vi "uc480_Flash_and_Trigger.vi"() -> ()   [LabVIEW 2016]
uses:
  D:/Fabrizio/Labview Projects/IR OPO Controller/Branches/Schwarzschild version/uc480DotNet.dll
  uc480DotNet.dll
panel:
  in  "Flash Duration":u32=10000
  in  "Flash Mode":string(combo)="0"
  in  "Trigger Mode":string(combo)="Software"
  out "Image":picture
  in  "Camera ID":i32 min=0 max=255
  out "Serial Number":string
  out "AOI Height":i32=8
  out "AOI Width":i32=8
  out "Bits/Pixel":i32=8
  out "Error Out":errorcluster caption="error"
  in  "Exit Camera":bool
  in  "Init Camera":bool
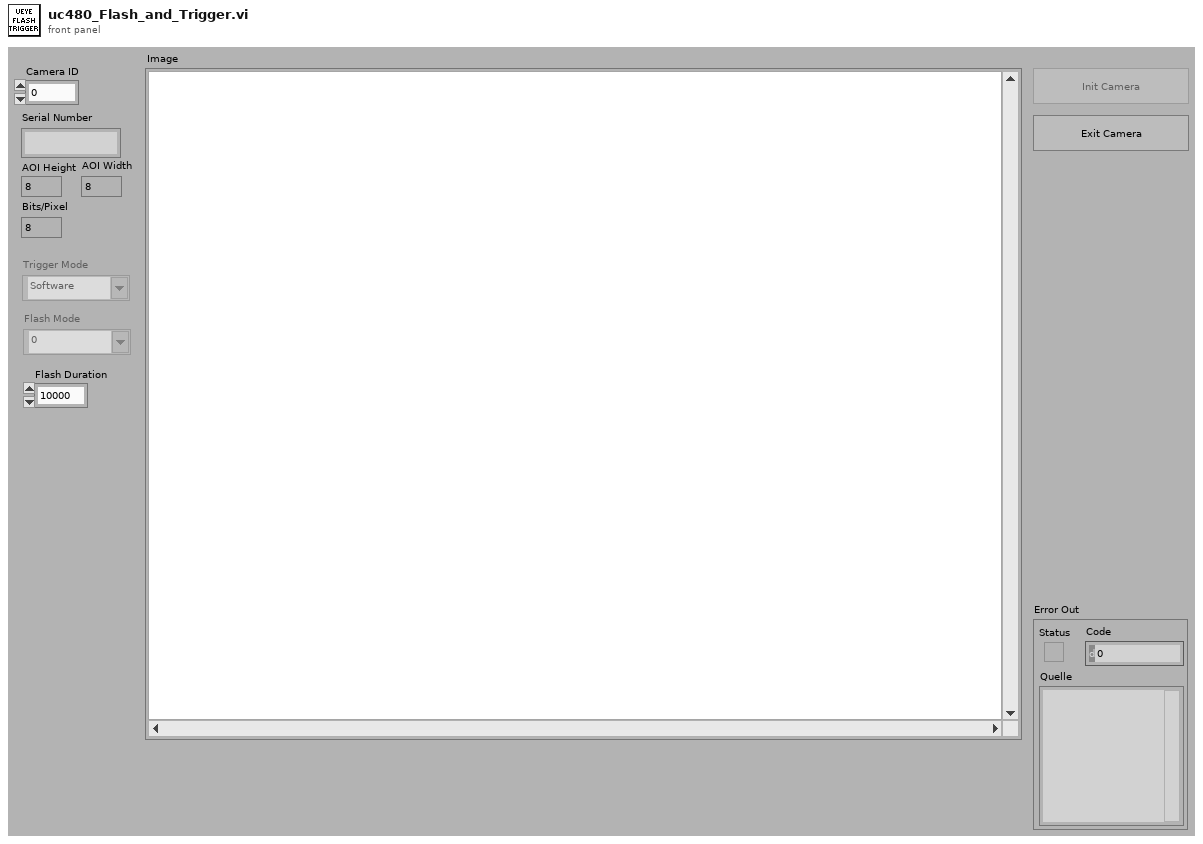
[diagram p1: front panel]
types:
  T1 = enum8{"Enabled", "Disabled", "Disabled and Grayed Out"}
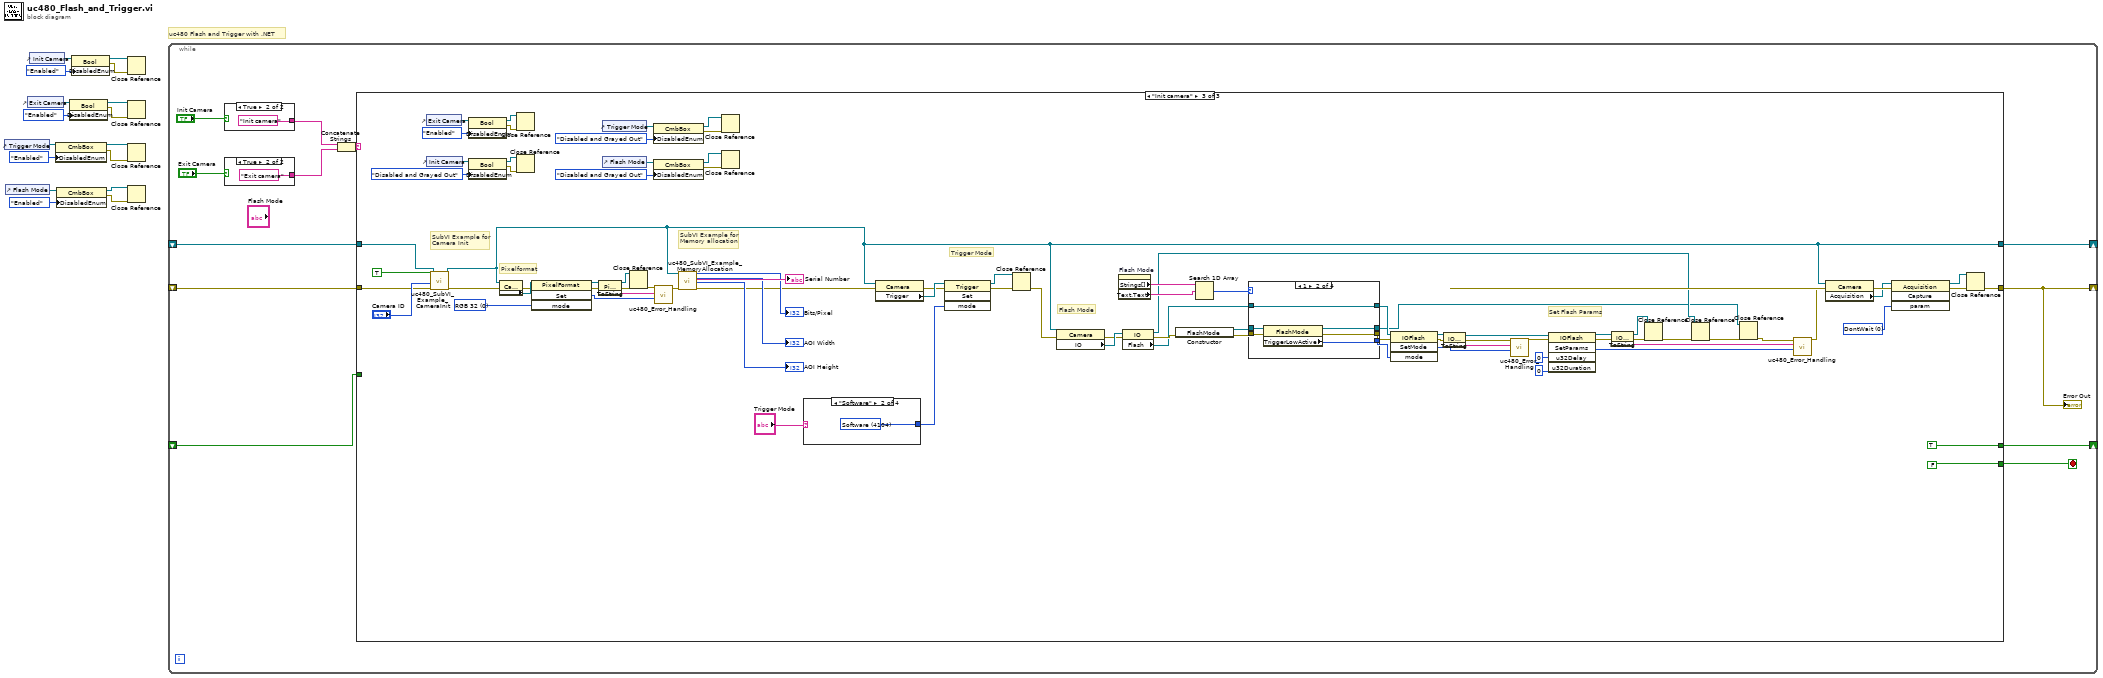
[diagram p0: block diagram]
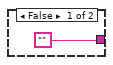
[diagram p2: hidden frame]
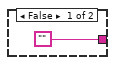
[diagram p3: hidden frame]
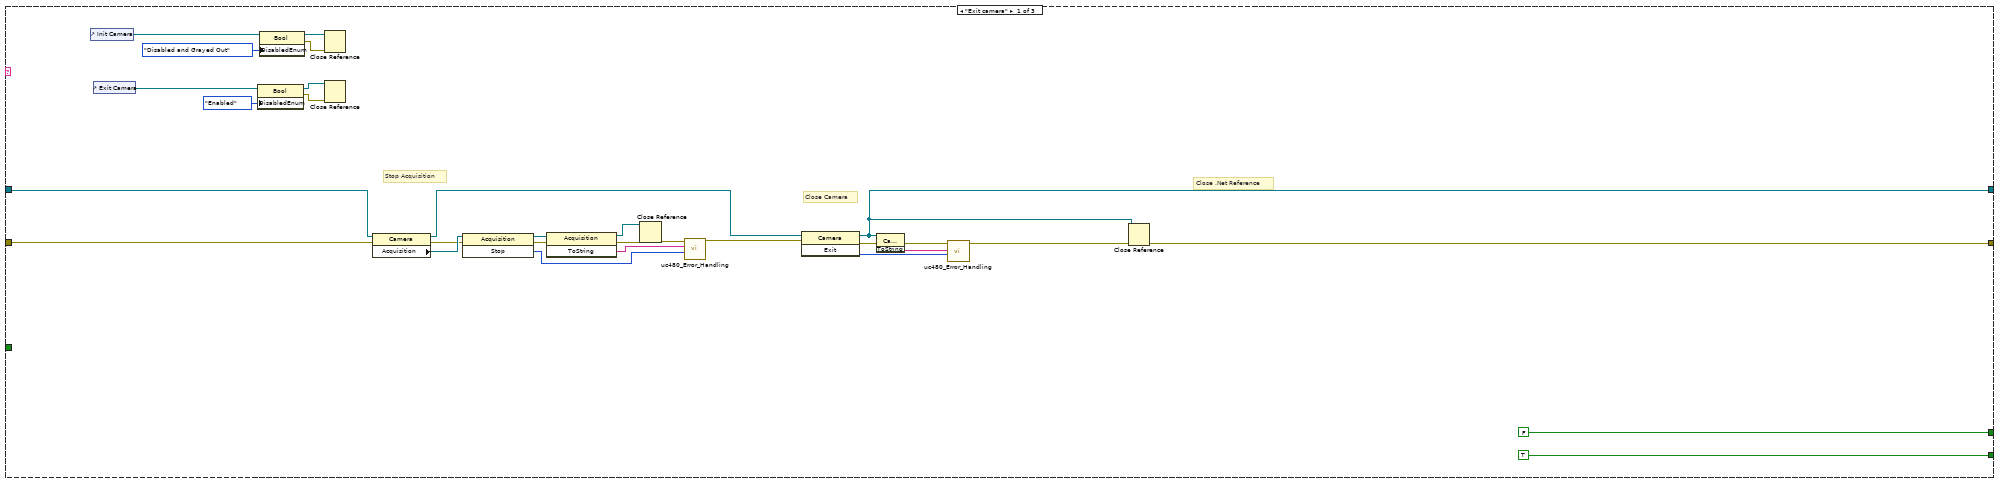
[diagram p4: hidden frame]
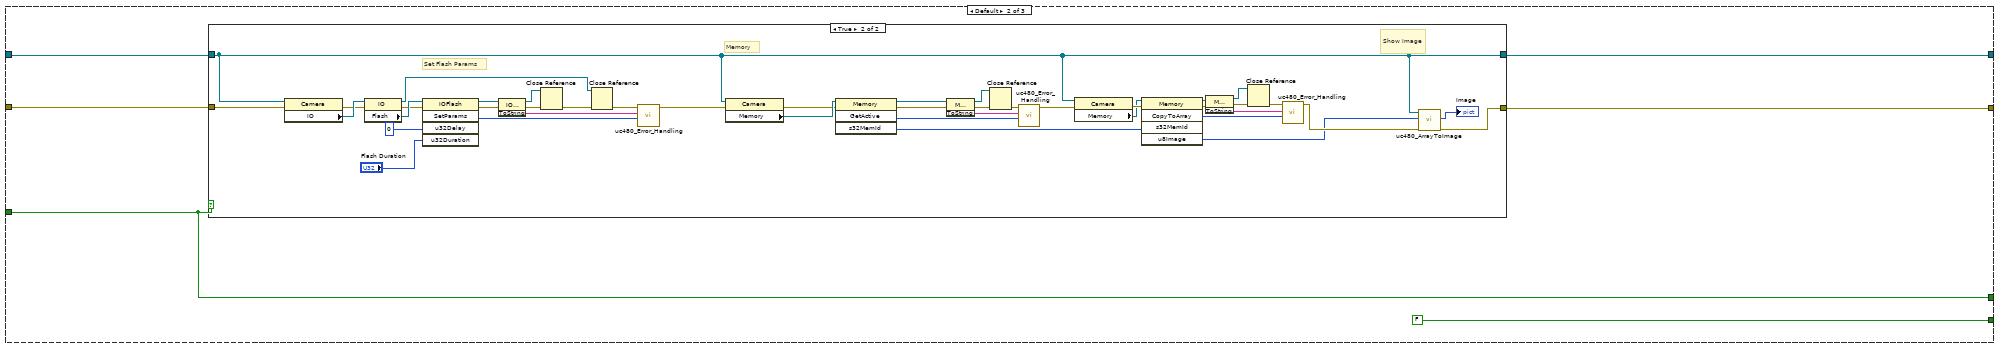
[diagram p5: hidden frame]
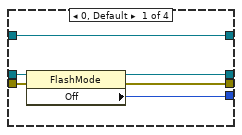
[diagram p7: hidden frame]
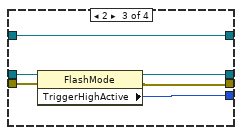
[diagram p8: hidden frame]
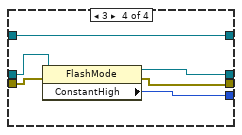
[diagram p9: hidden frame]
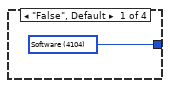
[diagram p10: hidden frame]
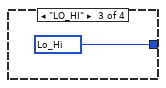
[diagram p11: hidden frame]
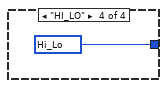
[diagram p12: hidden frame]
diagram:
  # "uc480 Flash and Trigger with .NET"
  n1 = control-ref of="Trigger Mode"() -> (w11:refnum<vi>)
  n2 = control-ref of="Flash Mode"() -> (w9:refnum<vi>)
  n3 = control-ref of="Exit Camera"() -> (w13:refnum<vi>)
  n4 = control-ref of="Init Camera"() -> (w14:refnum<vi>)
  n5 = property class="CmbBox"(reference=w11, "DisabledEnum"=T1."Enabled" ("Disabled")) -> (reference out=w5:refnum<vi>, error out=w6:errorcluster)  [unwired: 1 in]
  n6 = property class="CmbBox"(reference=w9, "DisabledEnum"=T1."Enabled" ("Disabled")) -> (reference out=w7:refnum<vi>, error out=w8:errorcluster)  [unwired: 1 in]
  n7 = property class="Bool"(reference=w13, "DisabledEnum"=T1."Enabled" ("Disabled")) -> (reference out=w3:refnum<vi>, error out=w4:errorcluster)  [unwired: 1 in]
  n8 = property class="Bool"(reference=w14, "DisabledEnum"=T1."Enabled" ("Disabled")) -> (reference out=w1:refnum<vi>, error out=w2:errorcluster)  [unwired: 1 in]
  n9 = Close Reference(reference=w1, error in (no error)=w2) -> ()  [unwired: 1 out]
  n10 = Close Reference(reference=w3, error in (no error)=w4) -> ()  [unwired: 1 out]
  n11 = Close Reference(reference=w5, error in (no error)=w6) -> ()  [unwired: 1 out]
  n12 = Close Reference(reference=w7, error in (no error)=w8) -> ()  [unwired: 1 out]
  n13 = while {
    shift-right: [w20] -> _
    shift-left: _ -> [w23]
    shift-right: [w22] -> _
    shift-left: _ -> [w17]
    shift-right: [w19] -> _
    shift-left: _ -> [w18]
    stop <- w21 stop-if-true
    n14 = case shown="True" "Init Camera" {
      tunnel: ["" "Init camera"] -> w27
      frame False {
      }
      frame True {
      }
    }
    n15 = case shown="True" "Exit Camera" {
      tunnel: ["" "Exit camera"] -> w24
      frame False {
      }
      frame True {
      }
    }
    n16 = Concatenate Strings(w27, w24) -> (w26:string)
    n17 = case shown="\"Init camera\"" w26 {
      tunnel: w17 -> [w38 w64 w190]
      tunnel: w23 -> [w47 w63 w189]
      tunnel: [w56 w66 w146] -> w22
      tunnel: [w55 w67 w128] -> w20
      tunnel: [TRUE FALSE FALSE] -> w21
      tunnel: [FALSE w65 TRUE] -> w19
      tunnel: w18 -> [_ w65 _]
      frame "Exit camera" {
        # "Close .Net Reference"
        # "Stop Acquisition"
        # "Close Camera"
        n18 = control-ref of="Init Camera"() -> (w43:refnum<vi>)
        n19 = control-ref of="Exit Camera"() -> (w42:refnum<vi>)
        n20 = property class="Bool"(reference=w42, "DisabledEnum"=T1."Enabled" ("Disabled")) -> (reference out=w33:refnum<vi>, error out=w34:errorcluster)  [unwired: 1 in]
        n21 = property class="Bool"(reference=w43, "DisabledEnum"=T1."Disabled and Grayed Out" ("Disabled")) -> (reference out=w35:refnum<vi>, error out=w36:errorcluster)  [unwired: 1 in]
        n22 = Close Reference(reference=w35, error in (no error)=w36) -> ()  [unwired: 1 out]
        n23 = Close Reference(reference=w33, error in (no error)=w34) -> ()  [unwired: 1 out]
        n24 = property class="Camera"(reference=w38, error in=w47) -> (reference out=w37:refnum<k24>, error out=w51:errorcluster, "Acquisition"=w52:refnum<k24>)
        n25 = invoke class="Acquisition" method="Stop"(reference=w52, error in=w51) -> (reference out=w49:refnum<k24>, error out=w50:errorcluster, "Stop"=w48:i32)  [unwired: 1 in]
        n26 = invoke class="Acquisition" method="ToString"(reference=w49, error in=w50) -> (reference out=w39:refnum<k24>, error out=w41:errorcluster, "ToString"=w53:string)  [unwired: 1 in]
        n27 = Close Reference(reference=w39, error in (no error)=w41) -> (error out=w40:errorcluster)
        n28 = call "uc480_Error_Handling.vi"("Error Code"=w48, "Error String"=w53, "Error In"=w40) -> ("Error Out"=w46:errorcluster)  [unwired: 8 in]
        n29 = invoke class="Camera" method="Exit"(reference=w37, error in=w46) -> (reference out=w56:refnum<k24>, error out=w59:errorcluster, "Exit"=w58:i32)  [unwired: 1 in]
        n30 = invoke class="Camera" method="ToString"(reference=w56, error in=w59) -> (error out=w60:errorcluster, "ToString"=w61:string)  [unwired: 1 in, 1 out]
        n31 = call "uc480_Error_Handling.vi"("Error Code"=w58, "Error String"=w61, "Error In"=w60) -> ("Error Out"=w57:errorcluster)  [unwired: 8 in]
        n32 = Close Reference ("Close Referenz")(reference=w56, error in (no error)=w57) -> (error out=w55:errorcluster)
      }
      frame Default {
        n33 = case shown="True" w65 {
          tunnel: [w70 w98] -> w67
          tunnel: w63 -> [w70 w83]
          tunnel: w64 -> [w69 w82]
          tunnel: [w69 w82] -> w66
          frame False {
          }
          frame True {
            # "Set Flash Params"
            # "Show Image"
            # "Memory"
            n34 = property on="Eigenschaftsknoten" class="Camera"(reference=w82, error in=w83) -> (error out=w89:errorcluster, "IO"=w91:refnum<k24>)  [unwired: 1 out]
            n35 = property on="Eigenschaftsknoten" class="IO"(reference=w91, error in=w89) -> (reference out=w77:refnum<k24>, error out=w90:errorcluster, "Flash"=w92:refnum<k24>)
            n36 = invoke class="IOFlash" method="SetParams"(reference=w92, error in=w90, "u32Delay"=u32 0 ("u32Duration"), "u32Duration"="Flash Duration") -> (reference out=w87:refnum<k24>, error out=w86:errorcluster, "SetParams"=w85:i32)  [unwired: 1 in, 2 out]
            n37 = invoke class="IOFlash" method="ToString"(reference=w87, error in=w86) -> (reference out=w80:refnum<k24>, error out=w81:errorcluster, "ToString"=w88:string)  [unwired: 1 in]
            n38 = Close Reference(reference=w80, error in (no error)=w81) -> (error out=w79:errorcluster)
            n39 = Close Reference(reference=w77, error in (no error)=w79) -> (error out=w78:errorcluster)
            n40 = call "uc480_Error_Handling.vi"("Error Code"=w85, "Error String"=w88, "Error In"=w78) -> ("Error Out"=w84:errorcluster)  [unwired: 8 in]
            n41 = property class="Camera"(reference=w82, error in=w84) -> (error out=w100:errorcluster, "Memory"=w101:refnum<k24>)  [unwired: 1 out]
            n42 = invoke class="Memory" method="GetActive"(reference=w101, error in=w100) -> (reference out=w106:refnum<k24>, error out=w105:errorcluster, "GetActive"=w107:i32, "s32MemId"=w99:i32)  [unwired: 2 in]
            n43 = invoke class="Memory" method="ToString"(reference=w106, error in=w105) -> (reference out=w74:refnum<k24>, error out=w76:errorcluster, "ToString"=w104:string)  [unwired: 1 in]
            n44 = Close Reference(reference=w74, error in (no error)=w76) -> (error out=w75:errorcluster)
            n45 = call "uc480_Error_Handling.vi"("Error Code"=w107, "Error String"=w104, "Error In"=w75) -> ("Error Out"=w108:errorcluster)  [unwired: 8 in]
            n46 = property class="Camera"(reference=w82, error in=w108) -> (error out=w103:errorcluster, "Memory"=w102:refnum<k24>)  [unwired: 1 out]
            n47 = invoke class="Memory" method="CopyToArray"(reference=w102, error in=w103, "s32MemId"=w99) -> (reference out=w110:refnum<k24>, error out=w111:errorcluster, "CopyToArray"=w112:i32, "u8Image"=w96:u8[])  [unwired: 2 in, 1 out]
            n48 = invoke class="Memory" method="ToString"(reference=w110, error in=w111) -> (reference out=w71:refnum<k24>, error out=w73:errorcluster, "ToString"=w109:string)  [unwired: 1 in]
            n49 = Close Reference(reference=w71, error in (no error)=w73) -> (error out=w72:errorcluster)
            n50 = call "uc480_Error_Handling.vi"("Error Code"=w112, "Error String"=w109, "Error In"=w72) -> ("Error Out"=w97:errorcluster)  [unwired: 8 in]
            n51 = call "uc480_ArrayToImage.vi"("Error In"=w97, "InArray"=w96, ".NET (Reference)"=w82) -> ("Error Out"=w98:errorcluster, "Image"=→"Image":picture)  [unwired: 7 in]
          }
        }
      }
      frame "Init camera" {
        w175 = 0 items=["DontWait"=0, "Wait"=1, "Force"=16384] ("param")
        w198 = 0 items=["RGB 32"=0, "RGB 24"=1, "Y8 Monochrom"=6] ("Mode")
        # "Trigger Mode"
        # "Set Flash Params"
        # "Flash Mode"
        # "SubVI Example for \nMemory allocation"
        # "SubVI Example for \nCamera Init"
        # "Pixelformat"
        n52 = control-ref of="Exit Camera"() -> (w169:refnum<vi>)
        n53 = control-ref of="Init Camera"() -> (w172:refnum<vi>)
        n54 = call <instrlib>:"uc480_SubVI_Example_CameraInit.vi"("Error In"=w189, "Camera ID"="Camera ID", "Init Camera Flag"=TRUE, ".NET (Reference)"=w190) -> ("Error Out"=w195:errorcluster, ".NET (Reference)"=w146:refnum<k24>)  [unwired: 6 in]
        n55 = property class="Bool"(reference=w169, "DisabledEnum"=T1."Enabled" ("Disabled")) -> (reference out=w119:refnum<vi>, error out=w120:errorcluster)  [unwired: 1 in]
        n56 = property class="Bool"(reference=w172, "DisabledEnum"=T1."Disabled and Grayed Out" ("Disabled")) -> (reference out=w117:refnum<vi>, error out=w118:errorcluster)  [unwired: 1 in]
        n57 = property class="Camera"(reference=w146, error in=w195) -> (error out=w196:errorcluster, "PixelFormat"=w197:refnum<k24>)  [unwired: 1 out]
        n58 = Close Reference(reference=w117, error in (no error)=w118) -> ()  [unwired: 1 out]
        n59 = Close Reference(reference=w119, error in (no error)=w120) -> ()  [unwired: 1 out]
        n60 = invoke class="PixelFormat" method="Set"(reference=w197, error in=w196, "mode"=w198) -> (reference out=w193:refnum<k24>, error out=w186:errorcluster, "Set"=w192:i32)  [unwired: 1 in, 1 out]
        n61 = invoke class="PixelFormat" method="ToString"(reference=w193, error in=w186) -> (reference out=w135:refnum<k24>, error out=w137:errorcluster, "ToString"=w194:string)  [unwired: 1 in]
        n62 = control-ref of="Trigger Mode"() -> (w167:refnum<vi>)
        n63 = control-ref of="Flash Mode"() -> (w140:refnum<vi>)
        n64 = Close Reference(reference=w135, error in (no error)=w137) -> (error out=w136:errorcluster)
        n65 = property class="CmbBox"(reference=w167, "DisabledEnum"=T1."Disabled and Grayed Out" ("Disabled")) -> (reference out=w116:refnum<vi>, error out=w115:errorcluster)  [unwired: 1 in]
        n66 = property class="CmbBox"(reference=w140, "DisabledEnum"=T1."Disabled and Grayed Out" ("Disabled")) -> (reference out=w114:refnum<vi>, error out=w113:errorcluster)  [unwired: 1 in]
        n67 = call "uc480_Error_Handling.vi"("Error Code"=w192, "Error String"=w194, "Error In"=w136) -> ("Error Out"=w181:errorcluster)  [unwired: 8 in]
        n68 = call <instrlib>:"uc480_SubVI_Example_MemoryAllocation.vi"(".NET (Reference)"=w146, "Error In"=w181) -> ("Bits/Pixel 2"=→"Bits/Pixel":i32, "Width"=→"AOI Width":i32, "Serial Number"=→"Serial Number":string, "Height"=→"AOI Height":i32, "Error Out"=w145:errorcluster)  [unwired: 13 in]
        n69 = Close Reference(reference=w116, error in (no error)=w115) -> ()  [unwired: 1 out]
        n70 = Close Reference(reference=w114, error in (no error)=w113) -> ()  [unwired: 1 out]
        n71 = case shown="\"Software\"" "Trigger Mode" {
          tunnel: [w223 w224 w225 w226] -> w173
          frame "False", Default {
            w223 = 4104 items=["Off"=0, "Hi_Lo_Sync"=16, "Lo_Hi_Sync"=32, "Continuous"=4096, "Hi_Lo"=4097, "Lo_Hi"=4098, "Software"=4104, "Hi_Lo_Pre"=4160, "Lo_Hi_Pre"=4224] ("mode")
          }
          frame "Software" {
            w224 = 4104 items=["Off"=0, "Hi_Lo_Sync"=16, "Lo_Hi_Sync"=32, "Continuous"=4096, "Hi_Lo"=4097, "Lo_Hi"=4098, "Software"=4104, "Hi_Lo_Pre"=4160, "Lo_Hi_Pre"=4224] ("mode")
          }
          frame "LO_HI" {
            w225 = 4098 items=["Off"=0, "Hi_Lo_Sync"=16, "Lo_Hi_Sync"=32, "Continuous"=4096, "Hi_Lo"=4097, "Lo_Hi"=4098, "Software"=4104, "Hi_Lo_Pre"=4160, "Lo_Hi_Pre"=4224] ("mode")
          }
          frame "HI_LO" {
            w226 = 4097 items=["Off"=0, "Hi_Lo_Sync"=16, "Lo_Hi_Sync"=32, "Continuous"=4096, "Hi_Lo"=4097, "Lo_Hi"=4098, "Software"=4104, "Hi_Lo_Pre"=4160, "Lo_Hi_Pre"=4224] ("mode")
          }
        }
        n72 = property class="Camera"(reference=w146, error in=w145) -> (error out=w179:errorcluster, "Trigger"=w180:refnum<k24>)  [unwired: 1 out]
        n73 = invoke class="Trigger" method="Set"(reference=w180, error in=w179, "mode"=w173) -> (reference out=w132:refnum<k24>, error out=w134:errorcluster)  [unwired: 1 in, 2 out]
        n74 = Close Reference(reference=w132, error in (no error)=w134) -> (error out=w133:errorcluster)
        n75 = property on="Eigenschaftsknoten" class="Camera"(reference=w146, error in=w133) -> (error out=w150:errorcluster, "IO"=w151:refnum<k24>)  [unwired: 1 out]
        n76 = property on="Flash Mode" class="CmbBox"() -> ("Strings[]"=w144:string[], "Text.Text"=w143:string)  [unwired: 2 in, 2 out]
        n77 = property on="Eigenschaftsknoten" class="IO"(reference=w151, error in=w150) -> (reference out=w124:refnum<k24>, error out=w164:errorcluster, "Flash"=w138:refnum<k24>)
        n78 = constructor class="FlashMode"(error in=w164) -> (reference out=w162:refnum<k24>, error out=w163:errorcluster)  [unwired: 2 in, 1 out]
        n79 = Search 1D Array(1D array=w144, element=w143) -> (index of element=w142:i32)  [unwired: 1 in]
        n80 = case shown="1" w142 {
          tunnel: w162 -> [w204 w209 w215 w220]
          tunnel: w163 -> [w203 w208 w214 w221]
          tunnel: w138 -> [w202 w210 w216 w219]
          tunnel: [w202 w210 w216 w219] -> w166
          tunnel: [w200 w206 w212 w218] -> w165
          tunnel: [w201 w207 w213 w222] -> w149
          tunnel: [w199 w205 w211 w217] -> w121
          frame 0, Default {
            n81 = property class="FlashMode"(reference=w204, error in=w203) -> (reference out=w199:refnum<k24>, error out=w200:errorcluster, "Off"=w201:i32)
          }
          frame 1 {
            n82 = property class="FlashMode"(reference=w209, error in=w208) -> (reference out=w205:refnum<k24>, error out=w206:errorcluster, "TriggerLowActive"=w207:i32)
          }
          frame 2 {
            n83 = property class="FlashMode"(reference=w215, error in=w214) -> (reference out=w211:refnum<k24>, error out=w212:errorcluster, "TriggerHighActive"=w213:i32)
          }
          frame 3 {
            n84 = property class="FlashMode"(reference=w220, error in=w221) -> (reference out=w217:refnum<k24>, error out=w218:errorcluster, "ConstantHigh"=w222:i32)
          }
        }
        n85 = invoke class="IOFlash" method="SetMode"(reference=w166, error in=w165, "mode"=w149) -> (reference out=w156:refnum<k24>, error out=w155:errorcluster, "SetMode"=w154:i32)  [unwired: 1 in, 1 out]
        n86 = invoke class="IOFlash" method="ToString"(reference=w156, error in=w155) -> (reference out=w126:refnum<k24>, error out=w152:errorcluster, "ToString"=w153:string)  [unwired: 1 in]
        n87 = call "uc480_Error_Handling.vi"("Error Code"=w154, "Error String"=w153, "Error In"=w152) -> ("Error Out"=w157:errorcluster)  [unwired: 8 in]
        n88 = invoke class="IOFlash" method="SetParams"(reference=w126, error in=w157, "u32Delay"=u32 0, "u32Duration"=u32 0) -> (reference out=w159:refnum<k24>, error out=w160:errorcluster, "SetParams"=w161:i32)  [unwired: 1 in, 2 out]
        n89 = invoke class="IOFlash" method="ToString"(reference=w159, error in=w160) -> (reference out=w130:refnum<k24>, error out=w131:errorcluster, "ToString"=w158:string)  [unwired: 1 in]
        n90 = Close Reference(reference=w130, error in (no error)=w131) -> (error out=w125:errorcluster)
        n91 = Close Reference(reference=w124, error in (no error)=w125) -> (error out=w123:errorcluster)
        n92 = Close Reference(reference=w121, error in (no error)=w123) -> (error out=w122:errorcluster)
        n93 = call "uc480_Error_Handling.vi"("Error Code"=w161, "Error String"=w158, "Error In"=w122) -> ("Error Out"=w147:errorcluster)  [unwired: 8 in]
        n94 = property class="Camera"(reference=w146, error in=w147) -> (error out=w177:errorcluster, "Acquisition"=w178:refnum<k24>)  [unwired: 1 out]
        n95 = invoke class="Acquisition" method="Capture"(reference=w178, error in=w177, "param"=w175) -> (reference out=w127:refnum<k24>, error out=w129:errorcluster)  [unwired: 1 in, 2 out]
        n96 = Close Reference(reference=w127, error in (no error)=w129) -> (error out=w128:errorcluster)
      }
    }
    "Error Out" <- w20
  }
